vi "Solve1.vi"(8 "Error In":errorcluster, 11 "object in":refnum<class "2024_9.lvclass">) -> (0 "Error Out":errorcluster, 2 "Result":u64, 3 "object out":refnum<class "2024_9.lvclass">)   [LabVIEW 2023, in "2024_9.lvclass"]
uses:
  2024_9.lvclass
  2024_9.lvclass/2024_9.ctl
panel:
  out "string 2":string
  out "ValueOfLastDiscData":i32
  out "IndexOfLastDiscData":i32
  out "string":string
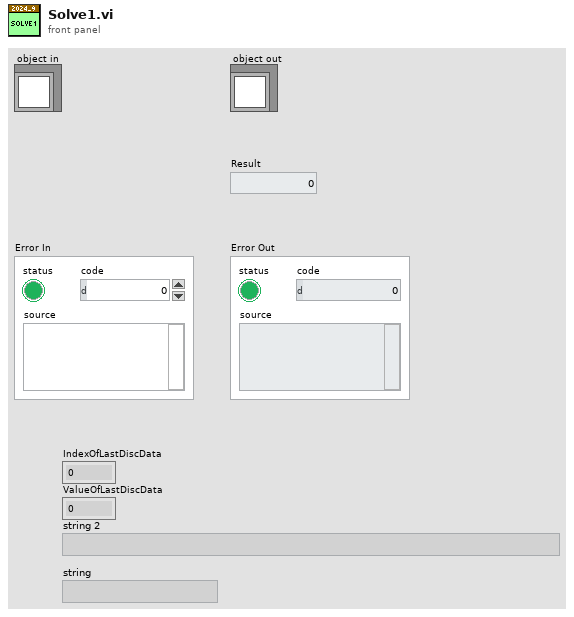
[diagram p1: front panel]
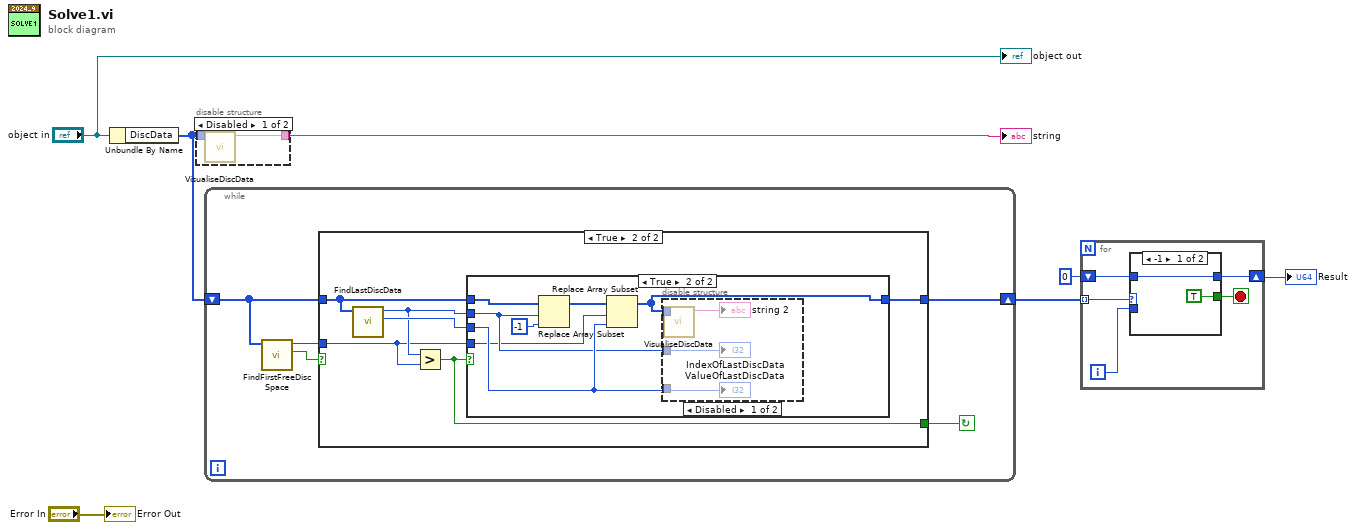
[diagram p0: block diagram]
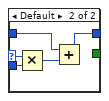
[diagram p3: hidden frame]
diagram:
  n1 = Unbundle By Name("object in") -> ("DiscData"=w4:i64[])
  n2 = disable-structure shown="Disabled" {
    disable-tunnel: [w9 _] -> w5
    disable-tunnel: w4 -> [w8 _]
    frame Disabled {
      n3 = call "VisualiseDiscData.vi"("DiscData"=w8) -> ("result string"=w9:string)  [unwired: 10 in]
    }
    frame Enabled {
    }
  }
  "string" <- w5
  n4 = while {
    shift-right: [w11] -> w3
    shift-left: w4 -> [w14]
    stop <- w10 continue-if-true
    n5 = call "FindFirstFreeDiscSpace.vi"("DiscData"=w14) -> ("FreeSpaceFound"=w12:bool, "IndexOfFirstFreeDiscSpace"=w13:i32)  [unwired: 9 in]
    n6 = case shown="True" w12 {
      tunnel: w14 -> [w15 w21]
      tunnel: w13 -> [_ w17]
      tunnel: [w15 w19] -> w11
      tunnel: [_ w16] -> w10
      frame False {
      }
      frame True {
        n7 = call "FindLastDiscData.vi"("DiscData"=w21) -> ("ValueOfLastDiscData"=w20:i64, "IndexOfLastDiscData"=w18:i32)  [unwired: 9 in]
        n8 = Greater?(x=w18, y=w17) -> (0:w16:bool)
        n9 = case shown="True" w16 {
          tunnel: w21 -> [w22 w29]
          tunnel: w20 -> [_ w26]
          tunnel: [w22 w25] -> w19
          tunnel: w18 -> [_ w24]
          tunnel: w17 -> [_ w23]
          frame False {
          }
          frame True {
            n10 = Replace Array Subset(array=w29, new element=i64 -1 ("new element/subarray"), index=w24) -> (w27:i64[])
            n11 = Replace Array Subset(array=w27, new element=w26, index=w23) -> (w25:i64[])
            n12 = disable-structure shown="Disabled" {
              disable-tunnel: w26 -> [w33 _]
              disable-tunnel: w25 -> [w31 _]
              disable-tunnel: w24 -> [w30 _]
              frame Disabled {
                n13 = call "VisualiseDiscData.vi"("DiscData"=w31) -> ("result string"=→"string 2":string)  [unwired: 10 in]
                "IndexOfLastDiscData" <- w30
                "ValueOfLastDiscData" <- w33
              }
              frame Enabled {
              }
            }
          }
        }
      }
    }
  }
  n14 = for {
    tunnel: w3 -> [w38] mode=indexing
    shift-right: [w35] -> w1
    shift-left: u64 0 -> [w36]
    i -> [w37]
    stop <- w34 stop-if-true
    n15 = case shown="-1" w38 {
      selector: w38 -> [_ w45]
      tunnel: w37 -> [_ w44]
      tunnel: w36 -> [w40 w42]
      tunnel: [w40 w41] -> w35
      tunnel: [TRUE _] -> w34
      frame -1 {
      }
      frame Default {
        n16 = Multiply(x=w45, y=w44) -> (x*y=w43:i64)
        n17 = Add(x=w42, y=w43) -> (x+y=w41:u64)
      }
    }
  }
  "Result" <- w1
  "Error Out" <- "Error In"
  "object out" <- "object in"
